vi "GeneratePoints.vi"(3 "N":dbl=250.0 format="%#_13g") -> (0 "(X, X^3)":cluster{dbl, dbl}[](array[cluster]), 1 "(X, X^2)":cluster{dbl, dbl}[](array[cluster]))   [LabVIEW 2013]
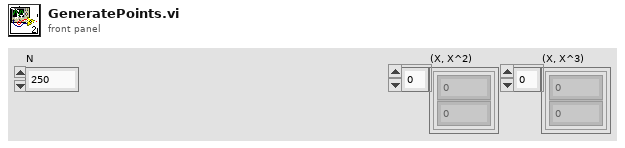
[diagram p1: front panel]
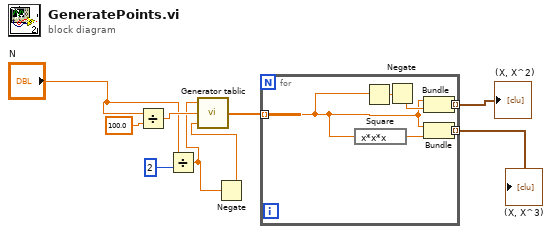
[diagram p0: block diagram]
diagram:
  n1 = Divide(x="N", y=100.0) -> (x/y=w8:dbl)
  n2 = Divide(x="N", y=u32 2) -> (x/y=w4:dbl)
  n3 = Negate(x=w4) -> (-x=w5:dbl)
  n4 = call "Generator tablic.vi"("Start"=w5, "Krok"=w8, "End"=w4) -> ("Array"=w7:dbl[])
  n5 = for {
    tunnel: w7 -> [w10] mode=indexing
    tunnel: [w12] -> w2 mode=indexing
    tunnel: [w11] -> w1 mode=indexing
    n6 = expression code="x*x*x"(w10) -> (w15:dbl)
    n7 = Square(x=w10) -> (x^2=w14:dbl)
    n8 = Negate(x=w14) -> (-x=w13:dbl)
    n9 = Bundle(w10, w13) -> (w12:cluster{dbl, dbl})  [unwired: 1 in]
    n10 = Bundle(w10, w15) -> (w11:cluster{dbl, dbl})  [unwired: 1 in]
  }
  "(X, X^2)" <- w2
  "(X, X^3)" <- w1
